vi "CHECK BARCODE AND CHECK.vi"(10 "BARCODE":string="02CRMTT1009190250KWPG", 11 "test sequence":path=path "D:/Configuration Folder Honda/config/test setting") -> (0 "Engine Prefix":string, 1 "Engine Model":string, 2 "Enum":T2=enum."Engine", 3 "MODEL":string, 7 "BARCODE 2":string="02CRMTT1009190250KWPG")   [LabVIEW 2015]
uses:
  Controls/BARCODE SELECTION.ctl
  test setting.ctl
  <vilib>/regexp/Match Regular Expression.xnode
panel:
  out "Array 2":bool[](array[boolean])
  out "offset past match":i32
  out "Model List":string[][](array[string])
  out "subarray":string[](array[string])
  out "substring 2":string
  out "Numeric":i32
  out "substring":string
  out "data":T1={"LCC"="02AHMSI1109190283LKWPG", "RCC"="02BHMSI1009190338RKWPG", "HEAD"="02CRMTT1009190250KWPG", "CRANK"="02BABCD1009190487LKWPG", "ENGINE"="02BABCD1009190487LKWPG", "BLOCK"="02CRMTT1009190250KWPG", "Setting 1"={"LCC"="02AHMSI1109190283LKWPG", "RCC"="02BHMSI1009190338RKWPG", "HEAD"="02CRMTT1009190250KWPG", "CRANK"="02BABCD1009190487LKWPG", "BLOCK"="02CRMTT1009190250KWPG"}, "Setting 2"={"LCC"="02AHMSI1109190283LKWPG", "RCC"="02BHMSI1009190338RKWPG", "HEAD"="02CRMTT1009190250KWPG", "CRANK"="02BABCD1009190487LKWPG", "BLOCK"="02CRMTT1009190250KWPG"}, "Model List"=[]}
  out "MODEL 2":string
  out "Array":bool[](array[boolean])
  in  "BLOCK":string="02BABCD1009190487LKWPG"
  out "number":u32
  in  "ENGINE":string="02BABCD1009190487LKWPG"
  in  "CRANK":string="02BABCD1009190487LKWPG"
  in  "HEAD":string="02CRMTT1009190250KWPG"
  in  "RCC":string="02BHMSI1009190338RKWPG"
  in  "LCC":string="02AHMSI1109190283LKWPG"
  # "Station 1"
  # "Station 2"
  # "Station 1"
  # "Station 2"
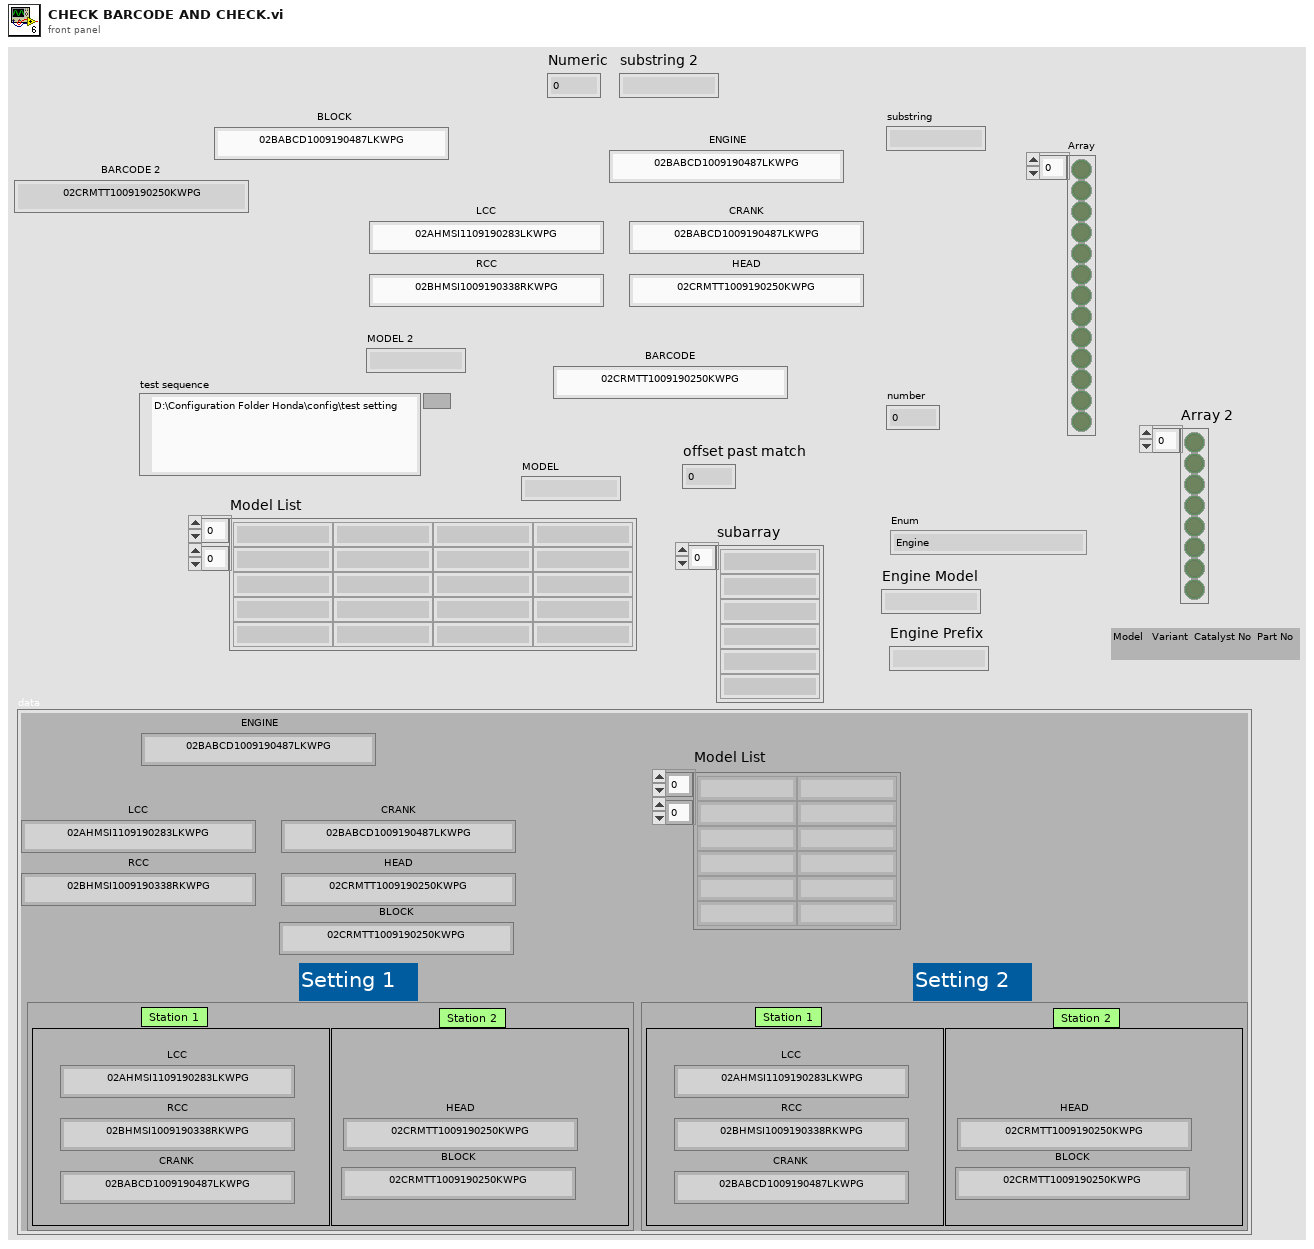
[diagram p1: front panel]
types:
  T1 = typedef "test setting.ctl" = cluster{"LCC":string, "RCC":string, "HEAD":string, "CRANK":string, "ENGINE":string, "BLOCK":string, "Setting 1":cluster{"LCC":string, "RCC":string, "HEAD":string, "CRANK":string, "BLOCK":string}, "Setting 2":cluster{"LCC":string, "RCC":string, "HEAD":string, "CRANK":string, "BLOCK":string}, "Model List":string[][]}
  T2 = typedef "BARCODE SELECTION.ctl" = enum16{"NO PART", "Engine", "LCC", "RCC", "HEAD", "BLOCK", "CRANK R", "CRANK L"}
  T3 = enum16{"open", "replace", "create", "open or create", "replace or create", "replace or create with confirmation"}
  T4 = cluster{"LCC":string, "RCC":string, "HEAD":string, "CRANK":string, "BLOCK":string}
  T5 = cluster{"LCC":string, "RCC":string, "HEAD":string, "CRANK":string, "BLOCK":string}[]
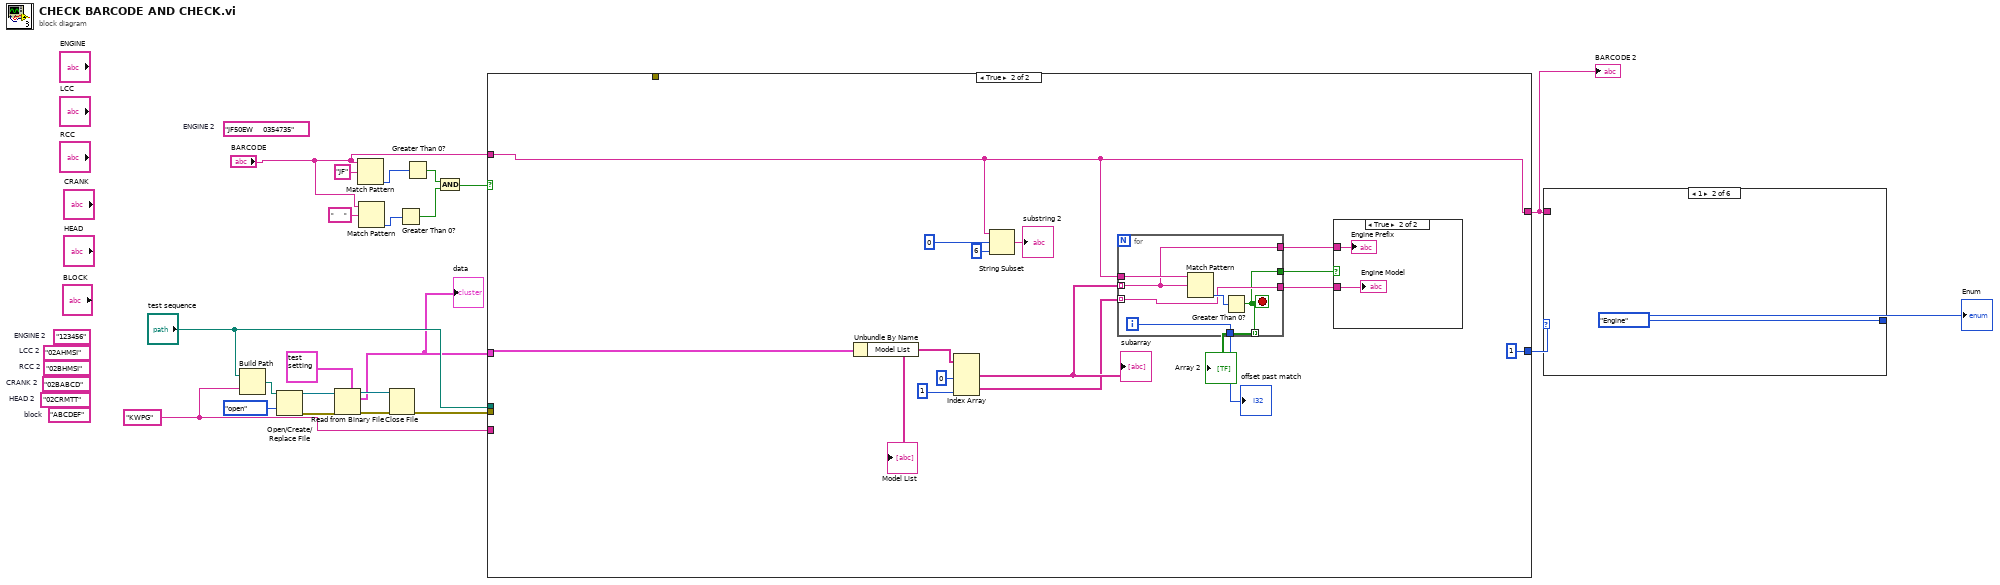
[diagram p0: block diagram]
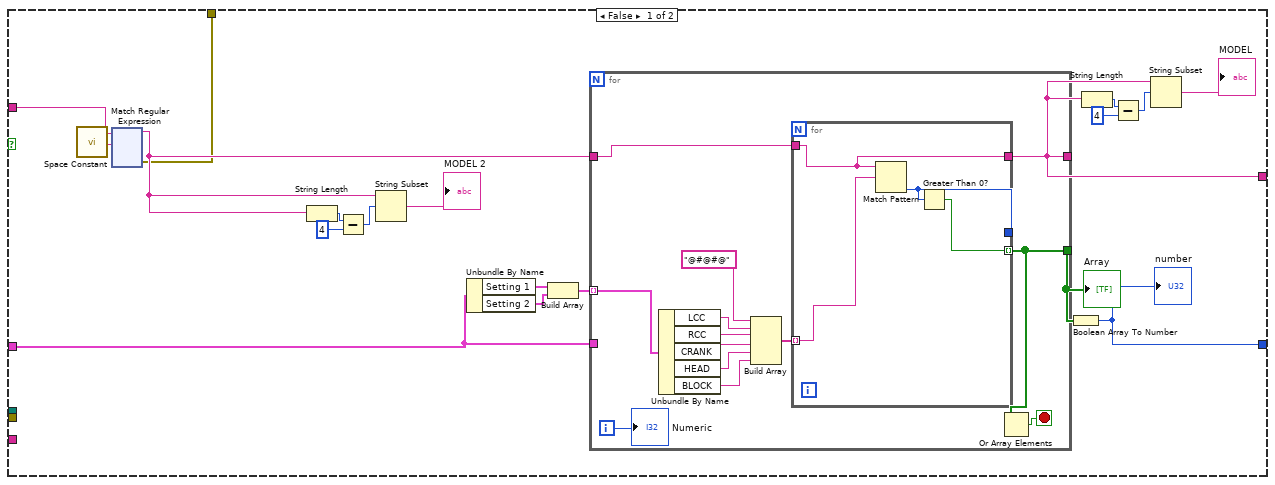
[diagram p2: hidden frame]
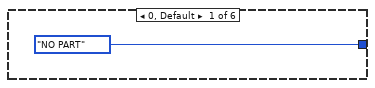
[diagram p4: hidden frame]
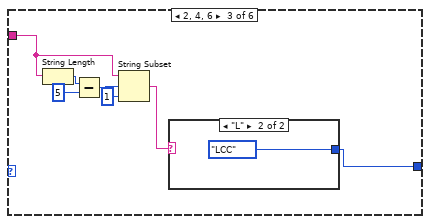
[diagram p5: hidden frame]
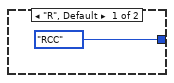
[diagram p6: hidden frame]
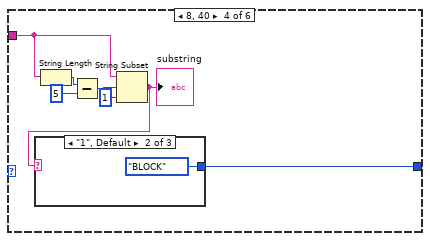
[diagram p7: hidden frame]
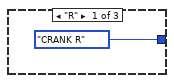
[diagram p8: hidden frame]
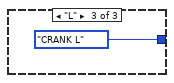
[diagram p9: hidden frame]
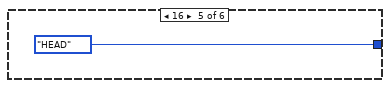
[diagram p10: hidden frame]
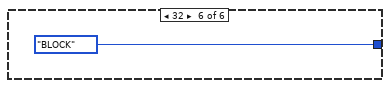
[diagram p11: hidden frame]
diagram:
  w4 = "KWPG" ("MODEL 3")
  (unwired) "JF50EW     0354735"  # ENGINE 2
  (unwired) "ABCDEF"  # block
  (unwired) "02CRMTT"  # HEAD 2
  (unwired) "02BABCD"  # CRANK 2
  (unwired) "02BHMSI"  # RCC 2
  (unwired) "02AHMSI"  # LCC 2
  (unwired) "123456"  # ENGINE 2
  n1 = Build Path(base path="test sequence", name or relative path=w4) -> (appended path=w10:path)
  n2 = Open/Create/Replace File(file path (use dialog)=w10, operation (0:open)=T3."open") -> (refnum out=w9:refnum<file>, error out=w8:errorcluster)  [unwired: 4 in, 1 out]
  n3 = Read from Binary File(5:T1 {"LCC"="", "RCC"="02BHMSI1009190338RKWPG", "HEAD"="02CRMTT1009190250KWPG", "CRANK"="", "ENGINE"="02BABCD1009190487LKWPG", "BLOCK"="02CRMTT1009190250KWPG", "Setting 1"={"LCC"="02AHMSI1109190283LKWPG", "RCC"="02BHMSI1009190338RKWPG", "HEAD"="02CRMTT1009190250KWPG", "CRANK"="02BABCD1009190487LKWPG", "BLOCK"="02CRMTT1009190250KWPG"}, "Setting 2"={"LCC"="02AHMSI1109190283LKWPG", "RCC"="02BHMSI1009190338RKWPG", "HEAD"="02CRMTT1009190250KWPG", "CRANK"="02BABCD1009190487LKWPG", "BLOCK"="02CRMTT1009190250KWPG"}, "Model List"=[]} ("Cluster"), 8:w8, 11:w9) -> (0:w6:errorcluster, 2:w1:T1, 3:w7:refnum<file>)  [unwired: 3 in, 1 out]
  "data" <- w1
  n4 = Match Pattern(string="BARCODE", regular expression="JF") -> (offset past match=w19:i32)  [unwired: 1 in, 3 out]
  n5 = Match Pattern(string="BARCODE", regular expression="     ") -> (offset past match=w20:i32)  [unwired: 1 in, 3 out]
  n6 = Close File(refnum=w7, error in=w6) -> (error out=w2:errorcluster)  [unwired: 1 out]
  n7 = Greater Than 0?(x=w20) -> (x > 0?=w15:bool)
  n8 = Greater Than 0?(x=w19) -> (x > 0?=w16:bool)
  n9 = And(x=w16, y=w15) -> (x .and. y?=w14:bool)
  n10 = case shown="True" w14 {
    tunnel: [w40 u32 1] -> w22
    tunnel: [w39 w181] -> w12
    tunnel: "BARCODE" -> [w30 w181]
    tunnel: [w25 _] -> _
    tunnel: w4 -> [_ _]
    tunnel: "test sequence" -> [_ _]
    tunnel: w1 -> [w23 w175]
    tunnel: w2 -> [_ _]
    frame False {
      n11 = call <vilib>:"Space Constant.vi"() -> ("String"=w31:string)
      n12 = xnode "Match Regular Expression"("input string"=w30, "regular expression"=w31) -> ("before match"=w29:string, "error out"=w25:errorcluster)  [unwired: 4 in, 3 out]
      n13 = String Length(string=w29) -> (length=w32:i32)
      n14 = Subtract(x=w32, y=4) -> (x-y=w34:i32)
      n15 = String Subset(string=w29, offset (0)=w34) -> (substring=→"MODEL 2":string)  [unwired: 1 in]
      n16 = Unbundle By Name(w23) -> ("Setting 1"=w28:T4, "Setting 2"=w27:T4)
      n17 = Build Array(w28, w27) -> (w26:T5)
      n18 = for {
        tunnel: [w44] -> w41
        tunnel: w23 -> [_]
        tunnel: w29 -> [w47]
        tunnel: [w53] -> w39
        tunnel: w26 -> [w46] mode=indexing
        i -> [w42]
        stop <- w43 stop-if-true
        n19 = Unbundle By Name(w46) -> ("LCC"=w52:string, "RCC"=w51:string, "CRANK"=w50:string, "HEAD"=w49:string, "BLOCK"=w48:string)
        n20 = Build Array("@#@#@" ("element"), w52, w51, w50, w49, w48) -> (w54:string[])
        n21 = for {
          tunnel: w47 -> [w55]
          tunnel: [w57] -> _
          tunnel: w54 -> [w58] mode=indexing
          tunnel: [w56] -> w44 mode=indexing
          tunnel: [w55] -> w53
          n22 = Match Pattern(string=w55, regular expression=w58) -> (offset past match=w57:i32)  [unwired: 1 in, 3 out]
          n23 = Greater Than 0?(x=w57) -> (x > 0?=w56:bool)
        }
        n24 = Or Array Elements(Boolean array=w44) -> (logical OR=w43:bool)
        "Numeric" <- w42
      }
      "Array" <- w41
      n25 = Boolean Array To Number(Boolean array=w41) -> (number=w40:u32)
      "number" <- w40
      n26 = String Length(string=w39) -> (length=w38:i32)
      n27 = Subtract(x=w38, y=4) -> (x-y=w36:i32)
      n28 = String Subset(string=w39, offset (0)=w36) -> (substring=→"MODEL":string)  [unwired: 1 in]
    }
    frame True {
      n29 = Unbundle By Name(w175) -> ("Model List"=w184:string[][])
      "Model List" <- w184
      n30 = Index Array(array=w184, index (col) #1=0 ("disabled index (col)"), index (col) #2=1 ("disabled index (col)")) -> (element #1=w182:string[], element #2=w178:string[])  [unwired: 2 in]
      "subarray" <- w182
      n31 = String Subset(string=w181, offset (0)=0, length (rest)=6 ("length (rest)")) -> (substring=→"substring 2":string)
      n32 = for {
        tunnel: w182 -> [w193] mode=indexing
        tunnel: w181 -> [w196]
        tunnel: [w194] -> w180
        tunnel: w178 -> [w192] mode=indexing
        tunnel: [w193] -> w177
        tunnel: [w192] -> w176
        tunnel: [w191] -> w174
        tunnel: [w191] -> w173 mode=indexing
        i -> [w194]
        stop <- w191 stop-if-true
        n33 = Match Pattern(string=w196, regular expression=w193) -> (offset past match=w195:i32)  [unwired: 1 in, 3 out]
        n34 = Greater Than 0?(x=w195) -> (x > 0?=w191:bool)
      }
      "offset past match" <- w180
      "Array 2" <- w173
      n35 = case shown="True" w174 {
        tunnel: w177 -> [_ w190]
        tunnel: w176 -> [_ w189]
        frame False {
        }
        frame True {
          "Engine Prefix" <- w190
          "Engine Model" <- w189
        }
      }
    }
  }
  "BARCODE 2" <- w12
  n36 = case shown="1" w22 {
    tunnel: [BARCODE_SELECTION."NO PART" BARCODE_SELECTION."Engine" w199 w214 BARCODE_SELECTION."HEAD" BARCODE_SELECTION."BLOCK"] -> w21
    tunnel: w12 -> [_ _ w200 w210 _ _]
    frame 0, Default {
    }
    frame 1 {
    }
    frame 2, 4, 6 {
      n37 = String Length(string=w200) -> (length=w202:i32)
      n38 = Subtract(x=w202, y=5) -> (x-y=w204:i32)
      n39 = String Subset(string=w200, offset (0)=w204, length (rest)=1 ("length (rest)")) -> (substring=w205:string)
      n40 = case shown="\"L\"" w205 {
        tunnel: [BARCODE_SELECTION."RCC" BARCODE_SELECTION."LCC"] -> w199
        frame "R", Default {
        }
        frame "L" {
        }
      }
    }
    frame 8, 40 {
      n41 = String Length(string=w210) -> (length=w211:i32)
      n42 = Subtract(x=w211, y=5) -> (x-y=w213:i32)
      n43 = String Subset(string=w210, offset (0)=w213, length (rest)=1 ("length (rest)")) -> (substring=w208:string)
      "substring" <- w208
      n44 = case shown="\"1\", Default" w208 {
        tunnel: [BARCODE_SELECTION."CRANK R" BARCODE_SELECTION."BLOCK" BARCODE_SELECTION."CRANK L"] -> w214
        frame "R" {
        }
        frame "1", Default {
        }
        frame "L" {
        }
      }
    }
    frame 16 {
    }
    frame 32 {
    }
  }
  "Enum" <- w21
